vi "FirstTest.vi"(8 "error in":errorcluster) -> (0 "error out":errorcluster, 2 "result":string, 3 "pass":bool)   [LabVIEW 2020, in "MeasurementServerTests.lvlib"]
uses:
  MeasurementServerTests.lvlib
  Runtime/MeasurementLink Session Management/Session Reservation/Connection.ctl
  Runtime/MeasurementLink Session Management/Session Reservation/Hardware Independent Connection.ctl
  Runtime/MeasurementLink Session Management/Session Reservation/Data.ctl
  Runtime/MeasurementLink Session Management Client/RPC Messages/ni_measurementlink_sessionmanagement_v1_SessionInformation.ctl
  Runtime/MeasurementLink Session Management Client/RPC Messages/nidevice_grpc_Session.ctl
  Runtime/MeasurementLink Session Management Client/RPC Messages/ni_measurementlink_sessionmanagement_v1_ChannelMapping.ctl
  8c161b2c-7580-4f71-9eec-17cc94e5f6f8.vi
  8c161b2c-7580-4f71-9eec-17cc94e5f6f8.vi/d089b476-b30c-4b91-b2ff-fbae0086b065.vi
  Runtime/MeasurementLink Session Management/Session Reservation/Get Connections Impl.vi
  <vilib>/Utility/error.llb/Error Cluster From Error Code.vi
  Runtime/MeasurementLink Session Management/Session Reservation/Session Reservation.lvclass
  Runtime/MeasurementLink Session Management Client/MeasurementLink Session Management Client.lvlib
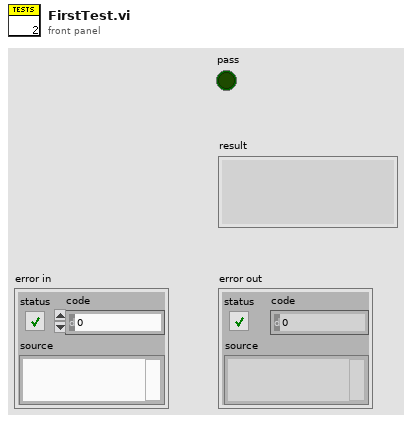
[diagram p1: front panel]
types:
  T1 = typedef "MeasurementLink Session Management Client.lvlib/ni_measurementlink_sessionmanagement_v1_ChannelMapping.ctl" = cluster{"pin_or_relay_name":string, "site":i32, "channel":string}
  T2 = typedef "MeasurementLink Session Management Client.lvlib/ni_measurementlink_sessionmanagement_v1_SessionInformation.ctl" = cluster{"session":T3, "resource_name":string, "channel_list":string, "instrument_type_id":string, "session_exists":bool, "channel_mappings":T1[]}
  T3 = typedef "MeasurementLink Session Management Client.lvlib/nidevice_grpc_Session.ctl" = cluster{"name":string}
  T4 = typedef "MeasurementLink Session Management.lvlib/Session Reservation.lvclass/Data.ctl" = cluster{"session infos":T2[], "sessions":variant[], "pins":string[]}
  T5 = typedef "MeasurementLink Session Management.lvlib/Session Reservation.lvclass/Connection.ctl" = cluster{"connection":T6, "session":variant}
  T6 = typedef "MeasurementLink Session Management.lvlib/Session Reservation.lvclass/Hardware Independent Connection.ctl" = cluster{"pin or relay name":string, "site":i32, "instrument type id":string, "channel":string}
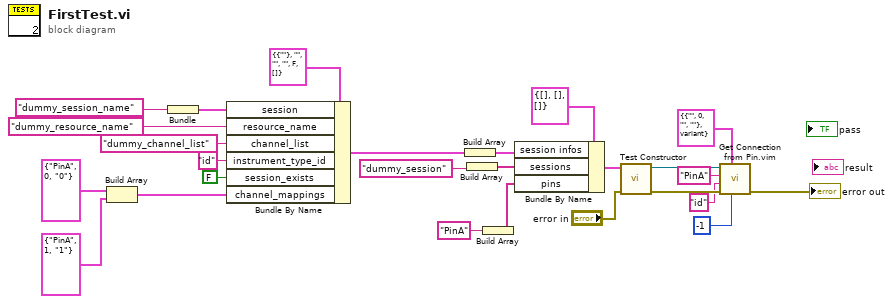
[diagram p0: block diagram]
diagram:
  n1 = Build Array(T1 {"pin_or_relay_name"="PinA", "site"=0, "channel"="0"} ("ni_measurementlink_sessionmanagement_v1_ChannelMapping"), T1 {"pin_or_relay_name"="PinA", "site"=1, "channel"="1"} ("ni_measurementlink_sessionmanagement_v1_ChannelMapping")) -> (w12:T1[])
  n2 = Bundle("dummy_session_name") -> (w18:cluster{string})  [unwired: 1 in]
  n3 = Bundle By Name(cluster=T2 {"session"={"name"=""}, "resource_name"="", "channel_list"="", "instrument_type_id"="", "session_exists"=FALSE, "channel_mappings"=[]} ("ni_measurementlink_sessionmanagement_v1_SessionInformation"), "session"=w18, "resource_name"="dummy_resource_name", "channel_list"="dummy_channel_list", "instrument_type_id"="id", "session_exists"=FALSE, "channel_mappings"=w12) -> (w21:T2)
  n4 = Build Array(w21) -> (w20:T2[])
  n5 = Build Array("dummy_session") -> (w11:string[])
  n6 = Build Array("PinA") -> (w9:string[])
  n7 = Bundle By Name(cluster=T4 {"session infos"=[], "sessions"=[], "pins"=[]} ("data"), "session infos"=w20, "sessions"=w11, "pins"=w9) -> (w8:T4)
  n8 = call "Test Constructor.vi"("error in"="error in", "data"=w8) -> ("error out"=w25:errorcluster, "Session Reservation out"=w24:refnum<class "Session Reservation.lvclass">)  [unwired: 8 in]
  n9 = call "Get Connection from Pin.vim"("site"=-1, "connection type"=T5 {"connection"={"pin or relay name"="", "site"=0, "instrument type id"="", "channel"=""}, "session"=variant} ("connection"), "error in"=w25, "instrument type id"="id", "pin or relay name"="PinA", "session reservation in"=w24) -> ("error out"=→"error out":errorcluster)  [unwired: 3 in, 2 out]
